vi "WPI_SafetyOutputVIRefnumList.vi"(0 "VI Refnum":refnum<vi>, 7 "menu":enum16{"read", "add", "remove"}(ring)) -> (4 "VI Refnums":refnum<vi>[](array[refnum]))   [LabVIEW 2017]
doc: "This holds the VI Refnums of the Safety Test VIs that will be called by the SafetyCheckEngine. All the VI Refnums must be strictly typed, so we can use the Call By Reference Node in the engine."
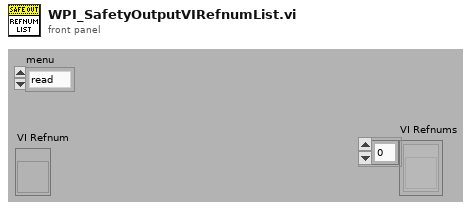
[diagram p1: front panel]
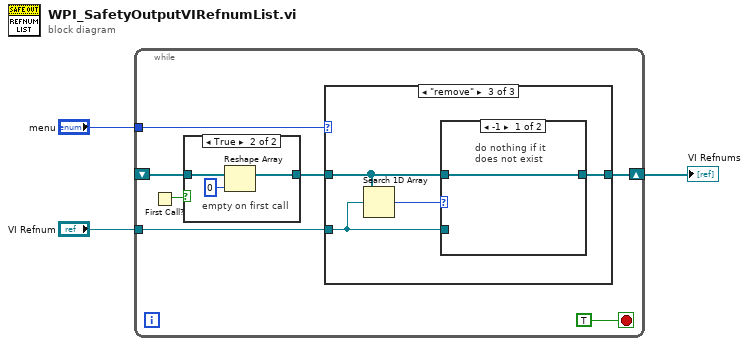
[diagram p0: block diagram]
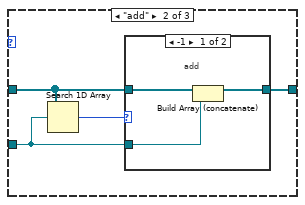
[diagram p4: hidden frame]
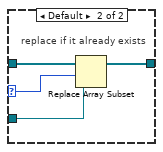
[diagram p5: hidden frame]
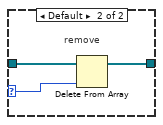
[diagram p6: hidden frame]
diagram:
  n1 = while {
    tunnel: "menu" -> [w9]
    tunnel: "VI Refnum" -> [w8]
    shift-right: [w7] -> w1
    shift-left: _ -> [w4]
    stop <- TRUE stop-if-true
    n2 = First Call?() -> (First Call?: T/F=w6:bool)
    n3 = case shown="True" w6 {
      tunnel: [w11 w13] -> w5
      tunnel: w4 -> [w11 w14]
      frame False {
      }
      frame True {
        # "empty on first call"
        n4 = Reshape Array(w14, 0 ("dimension size")) -> (w13:refnum<vi>[])
      }
    }
    n5 = case shown="\"remove\"" w9 {
      tunnel: w8 -> [_ w17 w28]
      tunnel: w5 -> [w15 w18 w29]
      tunnel: [w15 w19 w30] -> w7
      frame "read" {
      }
      frame "add" {
        n6 = Search 1D Array(1D array=w18, element=w17) -> (index of element=w16:i32)  [unwired: 1 out]
        n7 = case shown="-1" w16 {
          selector: w16 -> [_ w24]
          tunnel: w17 -> [w22 w23]
          tunnel: w18 -> [w21 w26]
          tunnel: [w20 w25] -> w19
          frame -1 {
            # "add"
            n8 = Build Array (concatenate)(w21, w22) -> (w20:refnum<vi>[])
          }
          frame Default {
            # "replace if it already exists"
            n9 = Replace Array Subset(array=w26, new element=w23, index=w24) -> (w25:refnum<vi>[])
          }
        }
      }
      frame "remove" {
        n10 = Search 1D Array(1D array=w29, element=w28) -> (index of element=w27:i32)  [unwired: 1 out]
        n11 = case shown="-1" w27 {
          selector: w27 -> [_ w32]
          tunnel: w28 -> [_ _]
          tunnel: w29 -> [w31 w34]
          tunnel: [w31 w33] -> w30
          frame -1 {
            # "do nothing if it does not exist"
          }
          frame Default {
            # "remove"
            n12 = Delete From Array(array=w34, index=w32) -> (array with subset deleted=w33:refnum<vi>[])  [unwired: 1 in, 1 out]
          }
        }
      }
    }
  }
  "VI Refnums" <- w1
